vi "InitiateClientHandshake.vi"(4 "remote port or service name":u16=7890, 6 "address":string="localhost", 7 "additional headers (none)":T1[](array[typedef]), 8 "error in (no error)":errorcluster, 9 "timeout ms (5000)":i32=5000, 11 "WebSocket Connection in":refnum<k5>) -> (0 "error out":errorcluster, 2 "Return Headers Out":variant, 3 "WebSocket Connection out":refnum<k5>)   [LabVIEW 2013, in "WebSockets.lvlib"]
doc: "Performs a client-side handshake. Sends the initial handshake HTTP header and waits for response from WebSocket server. Validates received accept key from the response."
uses:
  WebSockets.lvlib
  Headers.ctl
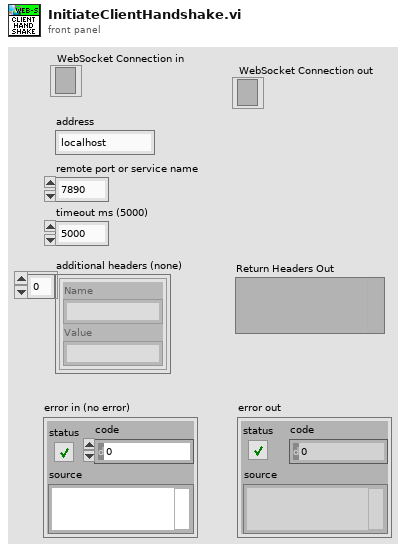
[diagram p1: front panel]
types:
  T1 = typedef "WebSockets.lvlib/Headers.ctl" = cluster{"Name":string, "Value":string}
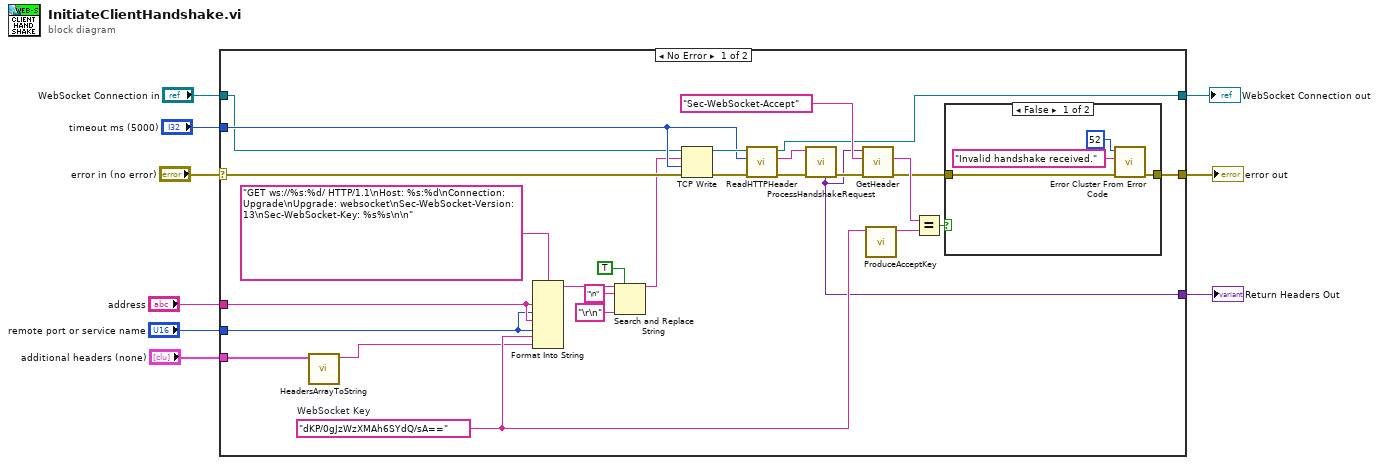
[diagram p0: block diagram]
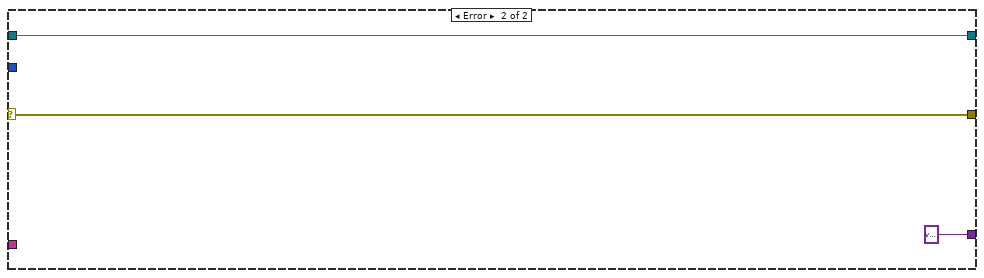
[diagram p3: hidden frame]
diagram:
  n1 = case shown="No Error" "error in (no error)" {
    selector: "error in (no error)" -> [w34 w44]
    tunnel: [w18 w43] -> w9
    tunnel: "WebSocket Connection in" -> [w14 w43]
    tunnel: [w15 w44] -> w6
    tunnel: "timeout ms (5000)" -> [w32 _]
    tunnel: [w20 variant ("Headers Out")] -> w4
    tunnel: "address" -> [w26 _]
    tunnel: "remote port or service name" -> [w25 _]
    tunnel: "additional headers (none)" -> [w11 _]
    frame No Error {
      w24 = "dKP/0gJzWzXMAh6SYdQ/sA=="  # WebSocket Key
      n2 = call "HeadersArrayToString.vi"("additional headers (none)"=w11) -> ("header string out"=w10:string)  [unwired: 10 in]
      n3 = Format Into String(format string="GET ws://%s:%d/ HTTP/1.1\nHost: %s:%d\nConnection: Upgrade\nUpgrade: websocket\nSec-WebSocket-Version: 13\nSec-WebSocket-Key: %s%s\n\n", w26, w25, w26, w25, w24, w10) -> (resulting string=w28:string)  [unwired: 2 in, 1 out]
      n4 = Search and Replace String(replace all?=TRUE ("replace all? (F)"), input string=w28, search string="\n", replace string="\r\n" ("replace string (\"\")")) -> (result string=w31:string)  [unwired: 4 in, 3 out]
      n5 = TCP Write(connection ID=w14, data in=w31, error in (no error)=w34, 9:w32) -> (connection ID out=w35:refnum<k5>, error out=w36:errorcluster)  [unwired: 1 out]
      n6 = call "ReadHTTPHeader.vi"("error in (no error)"=w36, "timeout ms (25000)"=w32, "WebSocket Connection in"=w35) -> ("error out"=w19:errorcluster, "HTTP Header"=w29:string, "WebSocket Connection out"=w18:refnum<k5>)  [unwired: 6 in]
      n7 = call "ProcessHandshakeRequest.vi"("error in (no error)"=w19, "HTTP Headers"=w29) -> ("error out"=w23:errorcluster, "Headers Out"=w20:variant)  [unwired: 4 in, 4 out]
      n8 = call "GetHeader.vi"("error in (no error)"=w23, "Name"="Sec-WebSocket-Accept", "Headers In"=w20) -> ("error out"=w16:errorcluster, "Data"=w21:string)  [unwired: 5 in, 2 out]
      n9 = call "ProduceAcceptKey.vi"("Sec-WebSocket-Key"=w24) -> ("Sec-WebSocket-Accept"=w30:string)  [unwired: 10 in]
      n10 = Equal?(x=w21, y=w30) -> (x = y?=w17:bool)
      n11 = case shown="False" w17 {
        tunnel: w16 -> [w39 w41]
        tunnel: [w40 w41] -> w15
        frame False {
          n12 = call <vilib>:"Error Cluster From Error Code.vi"("error in (no error)"=w39, "error message (\"\")"="Invalid handshake received." ("error message (\"\")"), "error code (0)"=52) -> ("error out"=w40:errorcluster)  [unwired: 6 in]
        }
        frame True {
        }
      }
    }
    frame Error {
    }
  }
  "WebSocket Connection out" <- w9
  "error out" <- w6
  "Return Headers Out" <- w4
